vi "PRM1Z8_Init.vi"(8 "error in (no error)":errorcluster) -> (0 "error out":errorcluster, 3 "reference out":refnum<k24>)   [LabVIEW 2018, in "Laser.lvlib"]
uses:
  Laser.lvlib
  C:/FlashGordon/Development/dll/ThorLabs.MotionControl.KCube.DCServoCLI.dll
  dll/ThorLabs.MotionControl.KCube.DCServoCLI.dll
  C:/FlashGordon/Development/dll/Thorlabs.MotionControl.DeviceManagerCLI.dll
  dll/Thorlabs.MotionControl.DeviceManagerCLI.dll
  C:/FlashGordon/Development/dll/Thorlabs.MotionControl.GenericMotorCLI.dll
  dll/Thorlabs.MotionControl.GenericMotorCLI.dll
panel:
  out "Controller Information":T1
  out "Device list (serial no.)":string[](array[string])
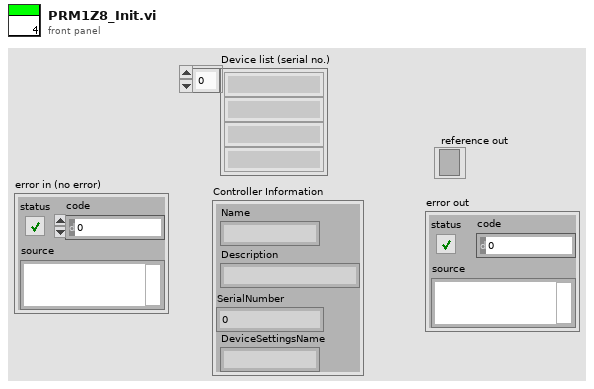
[diagram p1: front panel]
types:
  T1 = cluster{"Name":string, "Description":string, "SerialNumber":u32, "DeviceSettingsName":string}
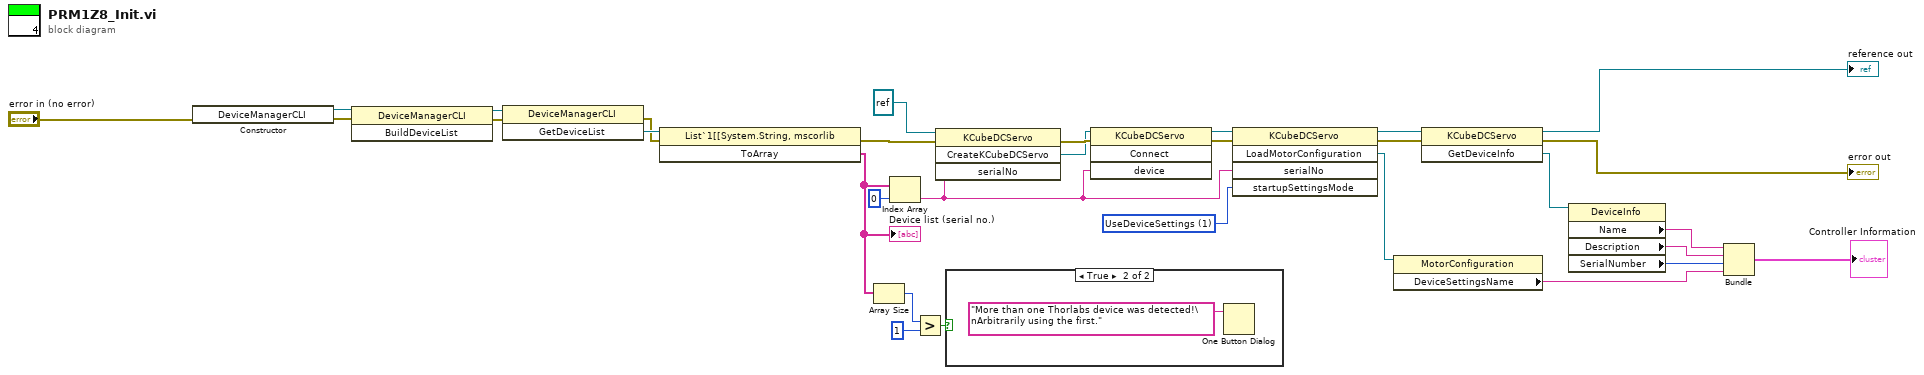
[diagram p0: block diagram]
diagram:
  w24 = 1 items=["UseDeviceSettings"=1, "UseFileSettings"=2, "UseConfiguredSettings"=3] ("startupSettingsMode")
  n1 = constructor class="DeviceManagerCLI"(error in="error in (no error)") -> (reference out=w5:refnum<k24>, error out=w6:errorcluster)  [unwired: 2 in, 1 out]
  n2 = invoke class="DeviceManagerCLI" method="BuildDeviceList"(reference=w5, error in=w6) -> (reference out=w19:refnum<k24>, error out=w21:errorcluster)  [unwired: 1 in, 1 out]
  n3 = invoke class="DeviceManagerCLI" method="GetDeviceList"(reference=w19, error in=w21) -> (error out=w18:errorcluster, "GetDeviceList"=w20:refnum<k24>)  [unwired: 1 in, 1 out]
  n4 = invoke class="List`1[[System.String, mscorlib" method="ToArray"(reference=w20, error in=w18) -> (error out=w17:errorcluster, "ToArray"=w4:string[])  [unwired: 1 in, 1 out]
  "Device list (serial no.)" <- w4
  n5 = Array Size(array=w4) -> (size(s)=w2:i32)
  n6 = Index Array(array=w4, index=0) -> (element=w15:string)
  n7 = Greater?(x=w2, y=1) -> (0:w3:bool)
  n8 = invoke class="KCubeDCServo" method="CreateKCubeDCServo"(reference=refnum<k24> refnum ("target class"), error in=w17, "serialNo"=w15) -> (error out=w26:errorcluster, "CreateKCubeDCServo"=w25:refnum<k24>)  [unwired: 1 in, 2 out]
  n9 = case shown="True" w3 {
    frame False {
    }
    frame True {
      n10 = One Button Dialog(message="More than one Thorlabs device was detected!\nArbitrarily using the first.") -> ()  [unwired: 1 in, 1 out]
    }
  }
  n11 = invoke class="KCubeDCServo" method="Connect"(reference=w25, error in=w26, "device"=w15) -> (reference out=w23:refnum<k24>, error out=w22:errorcluster)  [unwired: 1 in, 2 out]
  n12 = invoke class="KCubeDCServo" method="LoadMotorConfiguration"(reference=w23, error in=w22, "serialNo"=w15, "startupSettingsMode"=w24) -> (reference out=w9:refnum<k24>, error out=w8:errorcluster, "LoadMotorConfiguration"=w7:refnum<k24>)  [unwired: 1 in, 2 out]
  n13 = property class="MotorConfiguration"(reference=w7) -> ("DeviceSettingsName"=w14:string)  [unwired: 1 in, 2 out]
  n14 = invoke class="KCubeDCServo" method="GetDeviceInfo"(reference=w9, error in=w8) -> (reference out=→"reference out":refnum<k24>, error out=→"error out":errorcluster, "GetDeviceInfo"=w10:refnum<k24>)  [unwired: 1 in]
  n15 = property class="DeviceInfo"(reference=w10) -> ("Name"=w11:string, "Description"=w12:string, "SerialNumber"=w13:u32)  [unwired: 1 in, 2 out]
  n16 = Bundle("Name"=w11, "Description"=w12, "SerialNumber"=w13, "DeviceSettingsName"=w14) -> (→"Controller Information":T1)  [unwired: 1 in]
